vi "RT Main.vi"() -> ()   [LabVIEW 2021]
doc: "Demonstrates the use of Transmission Control Protocol (TCP) and meta data to receive messages from the host computer."
uses:
  <vilib>/myRIO/Express VI/Onboard Devices/LED/LED Express VI.xnode
  <vilib>/myRIO/Instrument Drivers/Onboard IO/DIO/vis/Write.vi
  <vilib>/myRIO/Instrument Drivers/Onboard IO/DIO/DIO.lvlib
  <vilib>/myRIO/Common/Instrument Driver Framework/myRIO v1.0/DIO/typedefs/DIO Channels Enum.ctl
  <vilib>/myRIO/Common/Instrument Driver Framework/myRIO v1.0/DIO/typedefs/DIO Channels List.ctl
  <vilib>/myRIO/Common/Instrument Driver Framework/Utilities/typedefs/Generic FPGA Reference.ctl
  <vilib>/myRIO/Common/Instrument Driver Framework/Utilities/typedefs/myRIO v1.0 Reference.ctl
  <vilib>/myRIO/Common/Instrument Driver Framework/Utilities/typedefs/Hardware Version Enum.ctl
  <vilib>/myRIO/Common/Instrument Driver Framework/Utilities/typedefs/myRIO Generic Hardware Reference.ctl
  <vilib>/myRIO/Instrument Drivers/Onboard IO/DIO/typedefs/DIO Reference.ctl
  <vilib>/myRIO/Instrument Drivers/Onboard IO/DIO/vis/myRIO DIO Open.xnode
  <vilib>/myRIO/Common/Instrument Driver Framework/Utilities/vis/Is FPGA Ref Available.vi
  <vilib>/myRIO/Common/Instrument Driver Framework/myRIO v1.0/DIO/vis/myRIO v1.1 Open DIO.vi
  <vilib>/userdefined/High Color/nirio_resource_hc.ctl
  <vilib>/myRIO/Instrument Drivers/Utilities/Utilities.lvlib
panel:
  out "LED Status":bool[](array[boolean])
  out "error out":errorcluster
  in  "Stop":bool
  in  "Host IP Address":string="172.22.11.1"
  # "Overview: Demonstrates the use of Transmission Control Protocol (TCP) and meta data to receive messages from the host computer.\nInstructions:\n1. Ensure Desktop Main.vi is already running.\n2. Verify the value in Host IP Address. If it is incorrect, specify the correct value.\n3. Observer the LEDs on the myRIO device and the value of LED Status on this VI. They change when the value of LED on Desktop Main.vi changes.\n4. Click Stop to stop this VI. Stopping this VI also terminates the running of Desktop Main.vi."
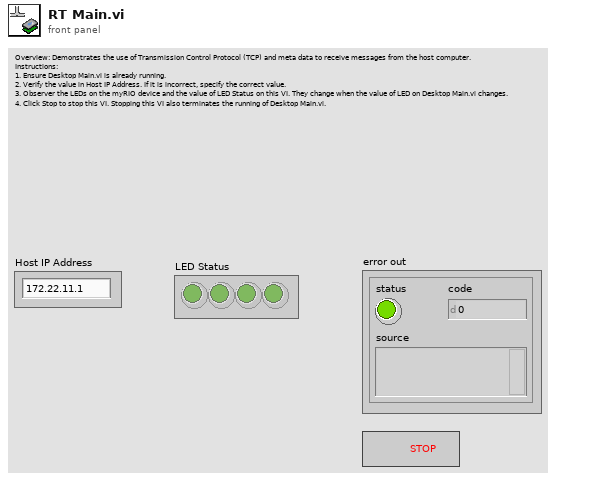
[diagram p1: front panel]
types:
  T1 = typedef "DIO.lvlib/DIO Reference.ctl" = cluster{"myRIO Reference":T2, "DIO Channels List":T6}
  T2 = typedef "myRIO Generic Hardware Reference.ctl" = cluster{"myRIO Model":T3, "myRIO Hardware Reference":T4}
  T3 = typedef "Hardware Version Enum.ctl" = enum16{"Unknown", "myRIO-1900", "myRIO-1950", "roboRIO", "NI ELVIS RIO CM", "ELVIS III"}
  T4 = typedef "myRIO v1.0 Reference.ctl" = cluster{"Generic FPGA Reference":T5, "Allow multiple opens":bool}
  T5 = typedef "Generic FPGA Reference.ctl" = refnum<k20>
  T6 = typedef "DIO Channels List.ctl" = T7[]
  T7 = typedef "DIO Channels Enum.ctl" = enum16{"Not Connected", "C/DIO0", "C/DIO1", "C/DIO2", "C/DIO3", "C/DIO4", "C/DIO5", "C/DIO6", "C/DIO7", "A/DIO0", "A/DIO1", "A/DIO2", "A/DIO3", "A/DIO4", "A/DIO5", "A/DIO6", "A/DIO7", "A/DIO8", "A/DIO9", "A/DIO10", "A/DIO11", "A/DIO12", "A/DIO13", "A/DIO14", "A/DIO15", "A/DIO16", "A/DIO17", "A/DIO18", "A/DIO19", "B/DIO0", "B/DIO1", "B/DIO2", "B/DIO3", "B/DIO4", "B/DIO5", "B/DIO6", "B/DIO7", "B/DIO8", "B/DIO9", "B/DIO10", "B/DIO11", "B/DIO12", "B/DIO13", "B/DIO14", "B/DIO15", "B/DIO16", "B/DIO17", "B/DIO18", "B/DIO19", "LED0", "LED1", "LED2", "LED3", "Button0", "DIO/DIO0", "DIO/DIO1", "DIO/DIO2", "DIO/DIO3", "DIO/DIO4", "DIO/DIO5", "DIO/DIO6", "DIO/DIO7", "DIO/DIO8", "DIO/DIO9", "SPI/CS0", "SPI/CS1", "SPI/CS2", "SPI/CS3", "LED RADIO (Green)", "LED RADIO (Red)", "LED COMM (Green)", "LED COMM (Red)", "LED MODE (Green)", "LED MODE (Red)"}
  T8 = typedef "nirio_resource_hc.ctl" = tag
  T9 = typedef "Connection Info.ctl" = cluster{"connection ID":refnum<k5>, "Meta data":string[]}
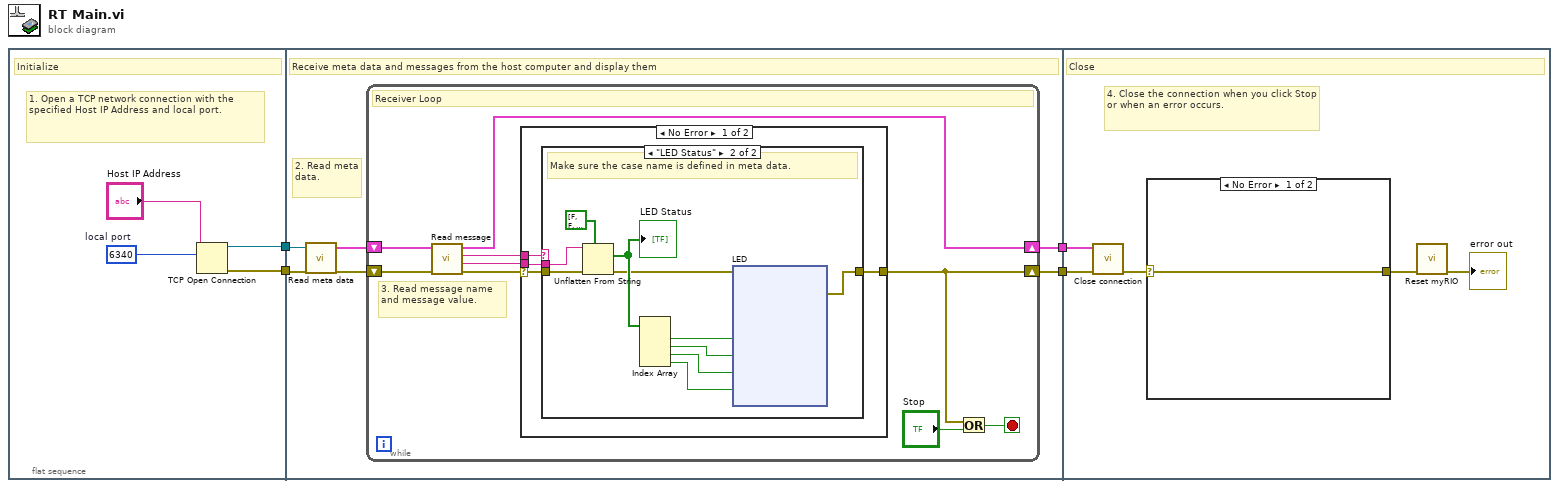
[diagram p0: block diagram]
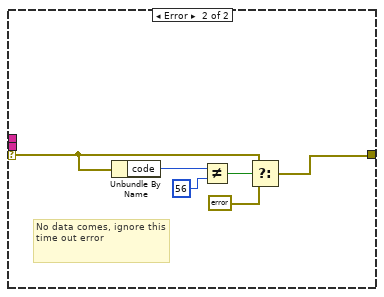
[diagram p3: hidden frame]
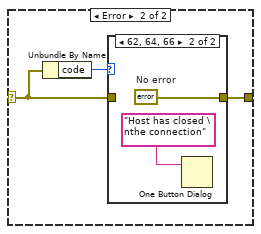
[diagram p4: hidden frame]
diagram:
  n1 = flat-sequence {
    tunnel: [w7] -> w2
    tunnel: [w6] -> w1
    tunnel: [w9] -> w4
    tunnel: [w10] -> w3
    tunnel: w2 -> [w14]
    tunnel: w1 -> [w13]
    tunnel: w4 -> [w87]
    tunnel: w3 -> [w86]
    frame #0 {
      w5 = u16 6340  # local port
      # "1. Open a TCP network connection with the specified Host IP Address and local port."
      # "Initialize"
      n2 = TCP Open Connection(address="Host IP Address", remote port or service name=w5) -> (connection ID=w7:refnum<k5>, error out=w6:errorcluster)  [unwired: 1 in, 2 out]
    }
    frame #1 {
      # "2. Read meta data."
      # "Receive meta data and messages from the host computer and display them"
      n3 = call "Read meta data.vi"("error in"=w13, "connection ID"=w14) -> ("error out"=w12:errorcluster, "Connection Info"=w11:T9)  [unwired: 8 in]
      n4 = while {
        shift-right: [w16] -> w10
        shift-left: w12 -> [w22]
        shift-right: [w15] -> w9
        shift-left: w11 -> [w23]
        stop <- w20 stop-if-true
        # "3. Read message name and message value."
        # "Receiver Loop"
        n5 = call "Read message.vi"("error in"=w22, "Connection Info"=w23) -> ("error out"=w19:errorcluster, "Messsage value"=w17:string, "Message name"=w18:string, "Connection Info out"=w15:T9)  [unwired: 6 in]
        n6 = case shown="No Error" w19 {
          selector: w19 -> [w25 w78]
          tunnel: [w24 w77] -> w16
          tunnel: w18 -> [w27 _]
          tunnel: w17 -> [w26 _]
          frame No Error {
            n7 = case shown="\"LED Status\"" w27 {
              tunnel: w26 -> [_ w38]
              tunnel: w25 -> [w28 w36]
              tunnel: [w28 w33] -> w24
              frame Default {
              }
              frame "LED Status" {
                # "Make sure the case name is defined in meta data."
                n8 = Unflatten From String(type=bool[] [FALSE, FALSE, FALSE, FALSE] ("LED Output"), binary string=w38, error in (no error)=w36) -> (value=w35:bool[], error out=w34:errorcluster)  [unwired: 3 out]
                "LED Status" <- w35
                n9 = Index Array(array=w35) -> (element #1=w32:bool, element #2=w31:bool, element #3=w30:bool, element #4=w29:bool)  [unwired: 4 in]
                n10 = xnode "LED"("LED0"=w32, "LED1"=w31, "LED2"=w30, "LED3"=w29, "error in (no error)"=w34) -> ("error out"=w33:errorcluster)
              }
            }
          }
          frame Error {
            # "No data comes, ignore this time out error"
            n11 = Unbundle By Name(w78) -> ("code"=w79:i32)
            n12 = Not Equal?(x=w79, y=56) -> (x != y?=w80:bool)
            n13 = Select(t=w78, s=w80, f=errorcluster {"status"=FALSE, "code"=0, "source"=""} ("error out")) -> (s? t:f=w77:errorcluster)
          }
        }
        n14 = Or(x=w16, y="Stop") -> (x .or. y?=w20:bool)
      }
    }
    frame #2 {
      # "4. Close the connection when you click Stop or when an error occurs."
      # "Close"
      n15 = call "Close connection.vi"("error in"=w86, "Connection Info"=w87) -> ("error out"=w85:errorcluster)  [unwired: 8 in, 1 out]
      n16 = case shown="No Error" w85 {
        selector: w85 -> [w88 w89]
        tunnel: [w88 w90] -> w84
        frame No Error {
        }
        frame Error {
          n17 = Unbundle By Name(w89) -> ("code"=w91:i32)
          n18 = case shown="62, 64, 66" w91 {
            tunnel: w89 -> [w92 _]
            tunnel: [w92 w93] -> w90
            frame Default {
            }
            frame 62, 64, 66 {
              w93 = errorcluster {"status"=FALSE, "code"=0, "source"=""}  # No error
              n19 = One Button Dialog(message="Host has closed \nthe connection") -> ()  [unwired: 1 in, 1 out]
            }
          }
        }
      }
      n20 = call <vilib>:"Reset myRIO.vi"("error in (no error)"=w84) -> ("error out"=→"error out":errorcluster)  [unwired: 10 in]
    }
  }
